vi "map_trap_switch.vi"() -> ()   [LabVIEW 2015]
panel:
  in  "ZeroLaser":bool
  in  "done":bool
  out "Mapping file":string
  in  "Done ?":bool
  in  "KILL":bool
  in  "PAUSE":bool
  in  "RESUME":bool
  in  "QUIT":bool
  in  "up done":bool
  in  "z up":bool
  in  "Done":bool
  in  "z piastra":bool
  in  "x piastra":bool
  in  "goto y pos":bool
  in  "goto x pos":bool
  in  "Panello o pcb?":bool
  in  "End":bool
  in  "zero z - end":bool
  in  "zero x - end":bool
  in  "zero y - end":bool
  in  "positioning done":bool
  out "output":string
  out "command":string
  in  "zero done":bool
  in  "zero z":bool
  in  "zero x":bool
  in  "zero y":bool
  # "Comandi di emergenza"
  # "In alto: TRUE ---> Panello"
  # "In basso: FALSE ---> PCB"
  # "Posiziono in zero"
  # "Vado sulla piastra \ne azzero"
  # "Azzero  il laser"
  # "Alzo il laser"
  # "Vado in posizione"
  # "Ritorno a zero"
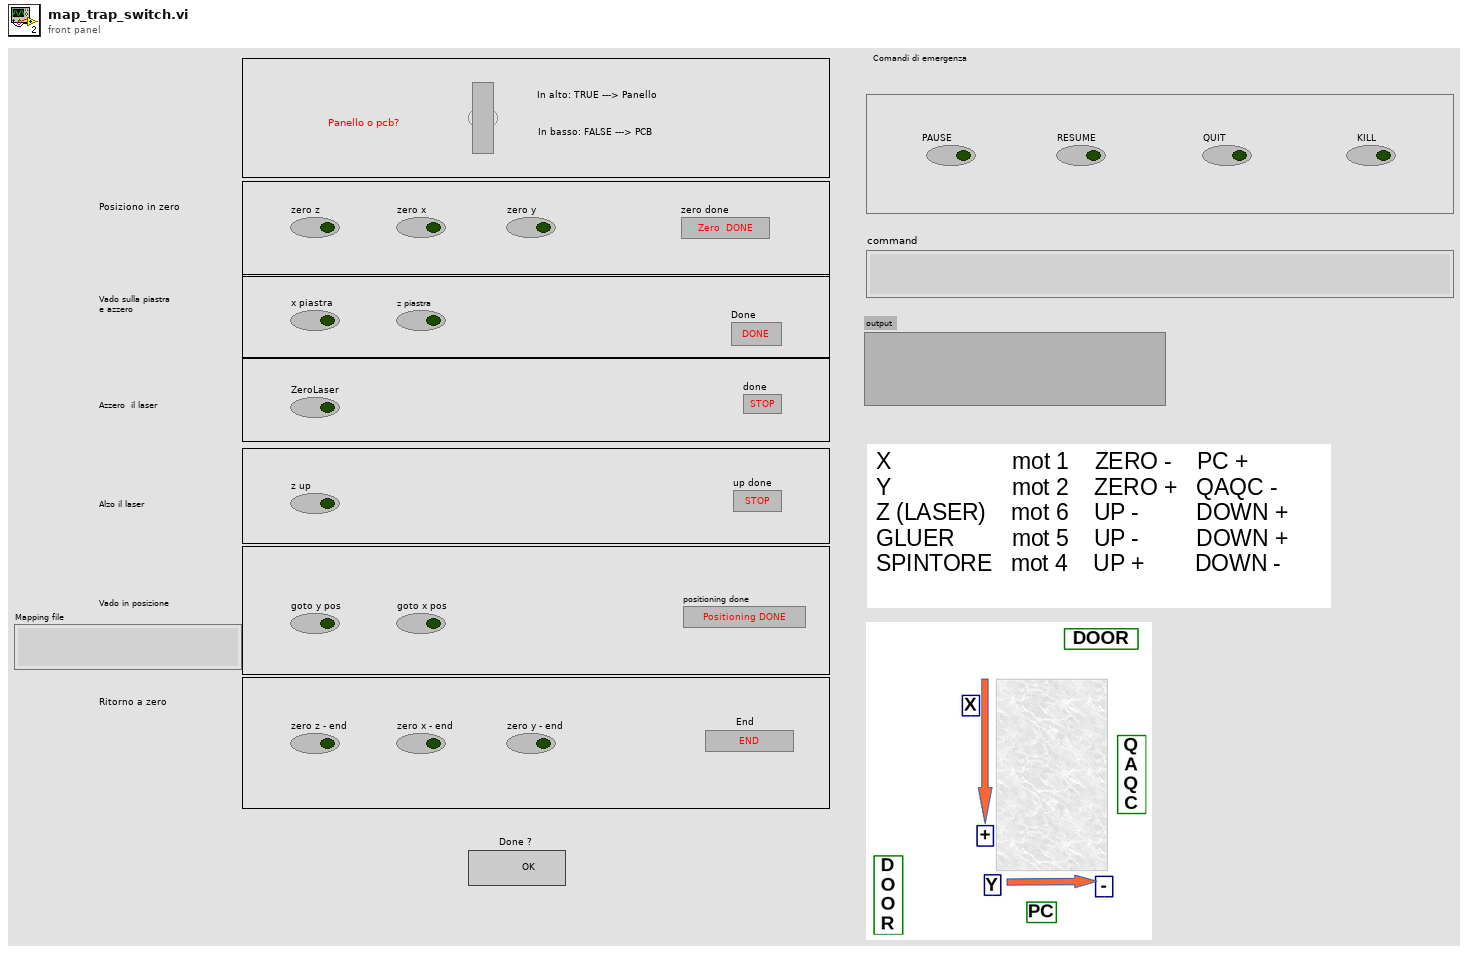
[diagram p1: front panel]
types:
  T1 = enum16{"open", "replace", "create", "open or create", "replace or create", "replace or create with confirmation"}
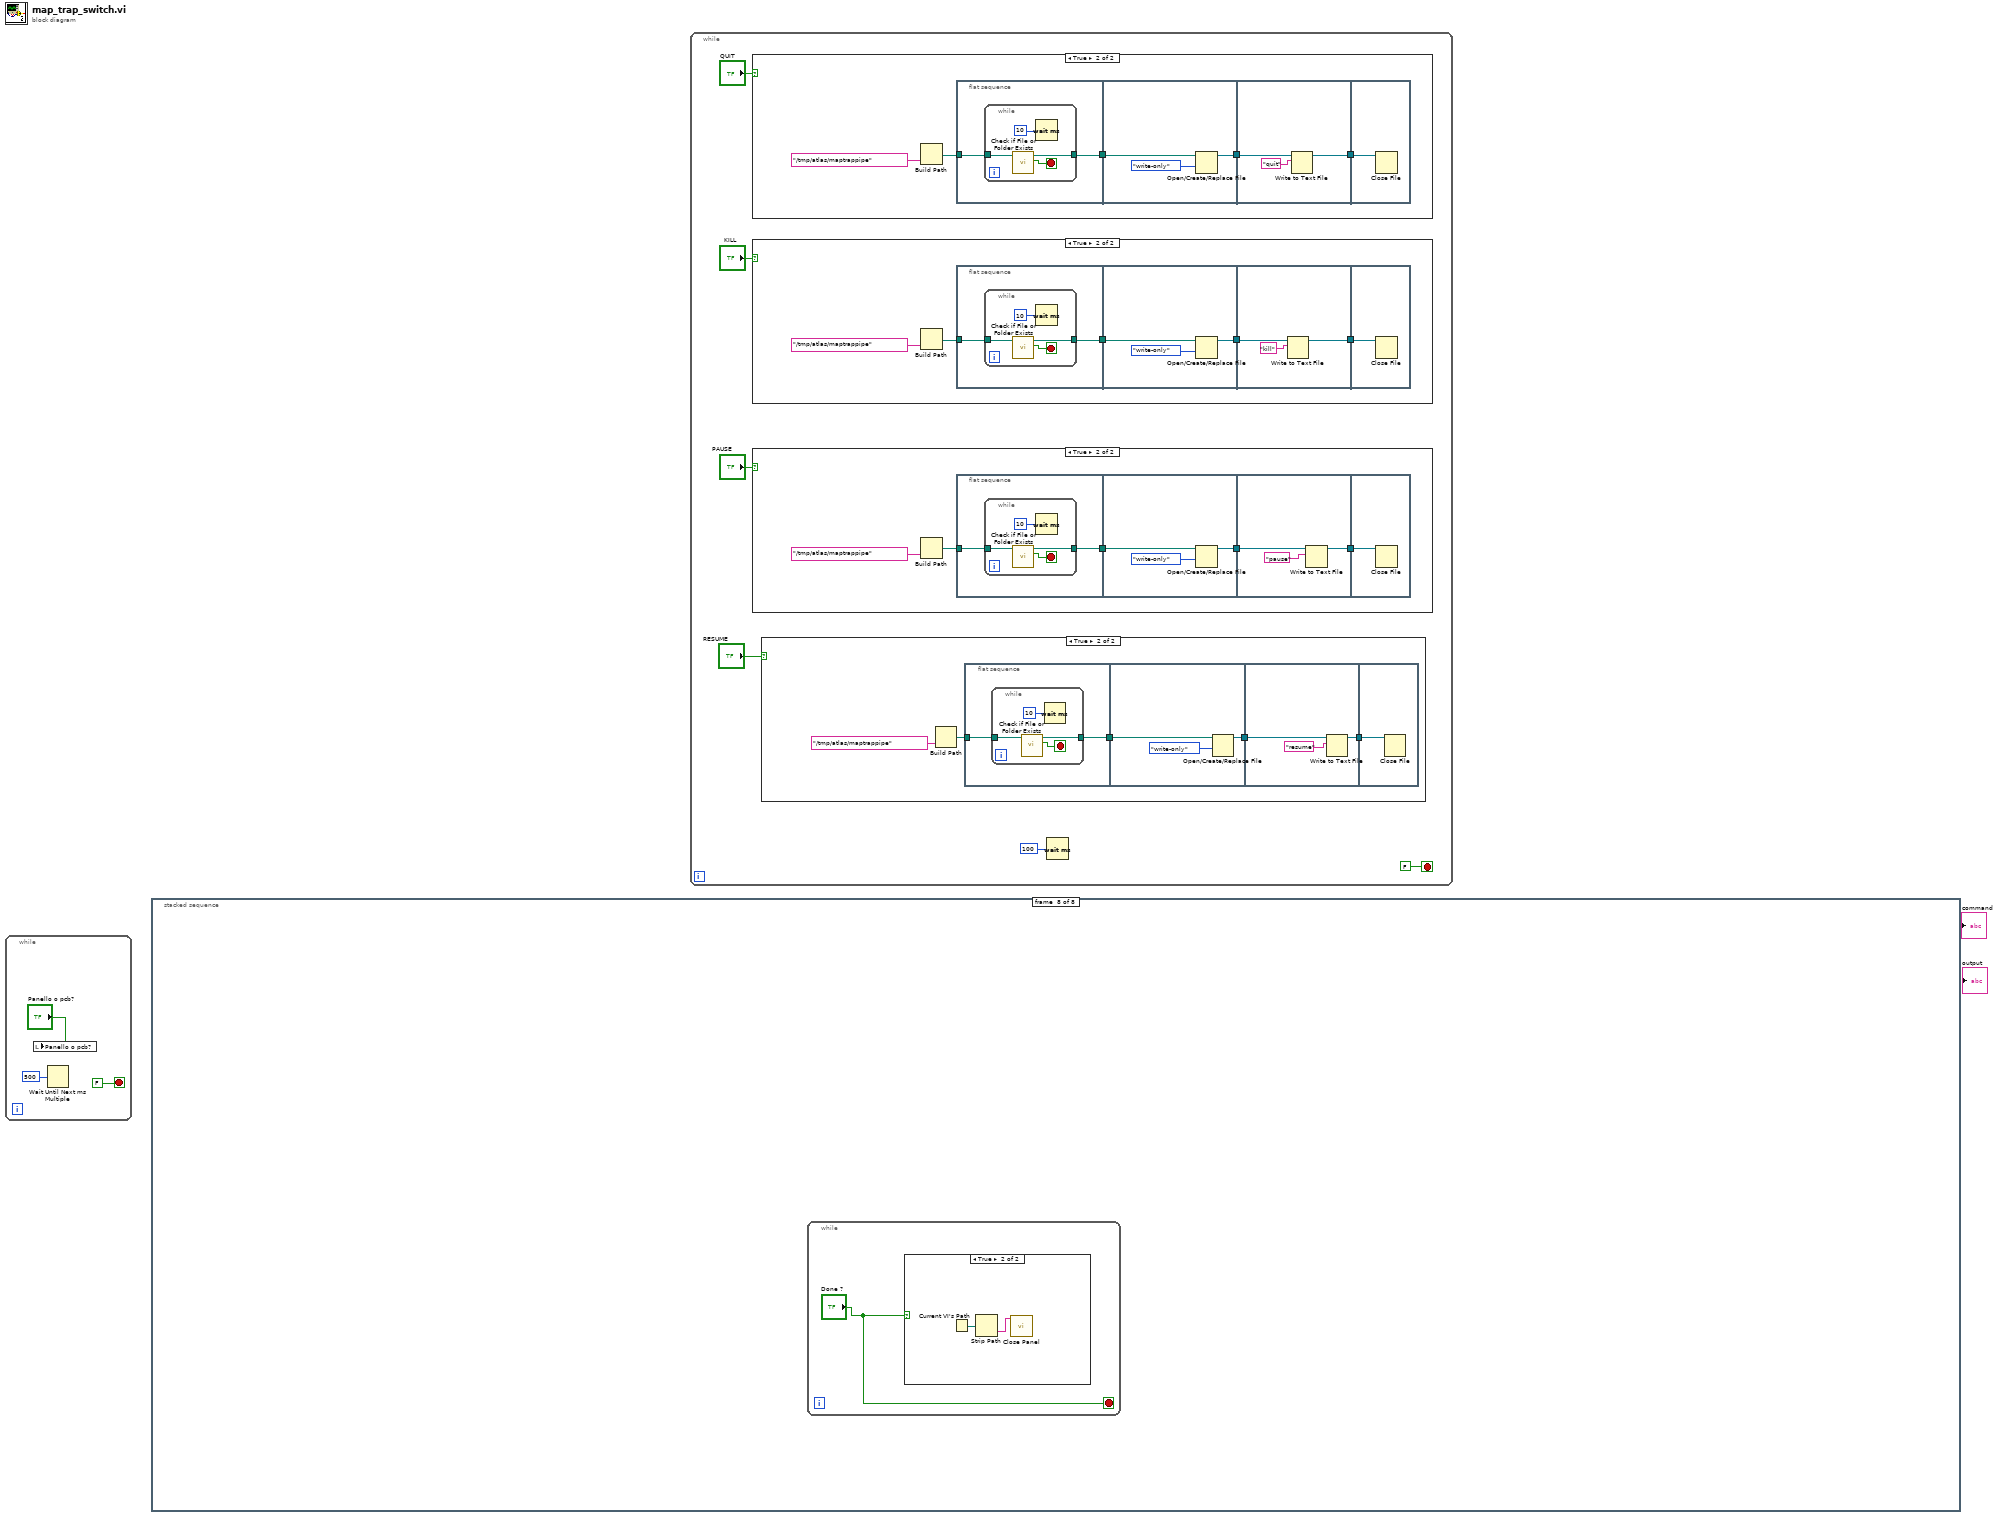
[diagram p0: block diagram]
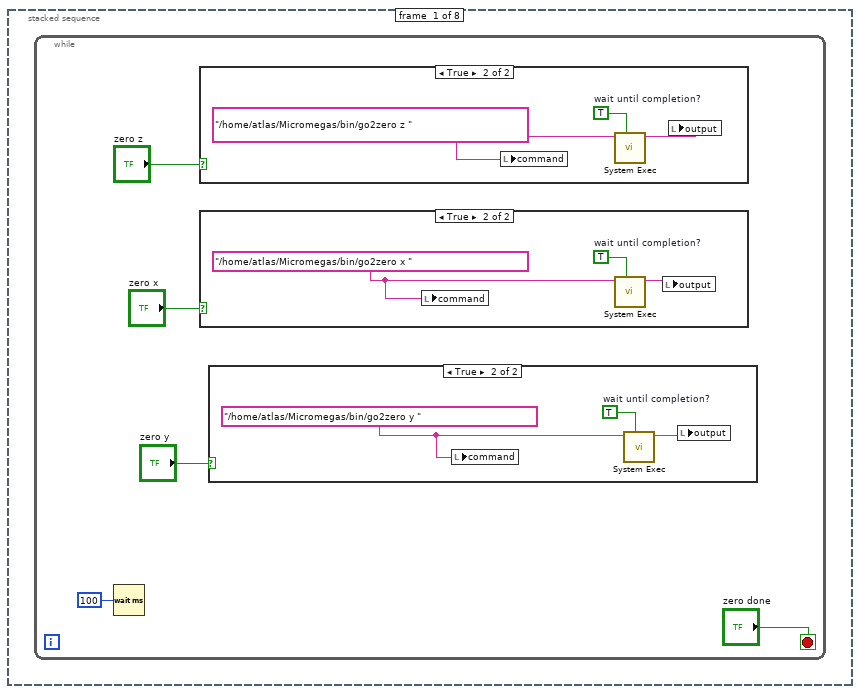
[diagram p6: hidden frame]
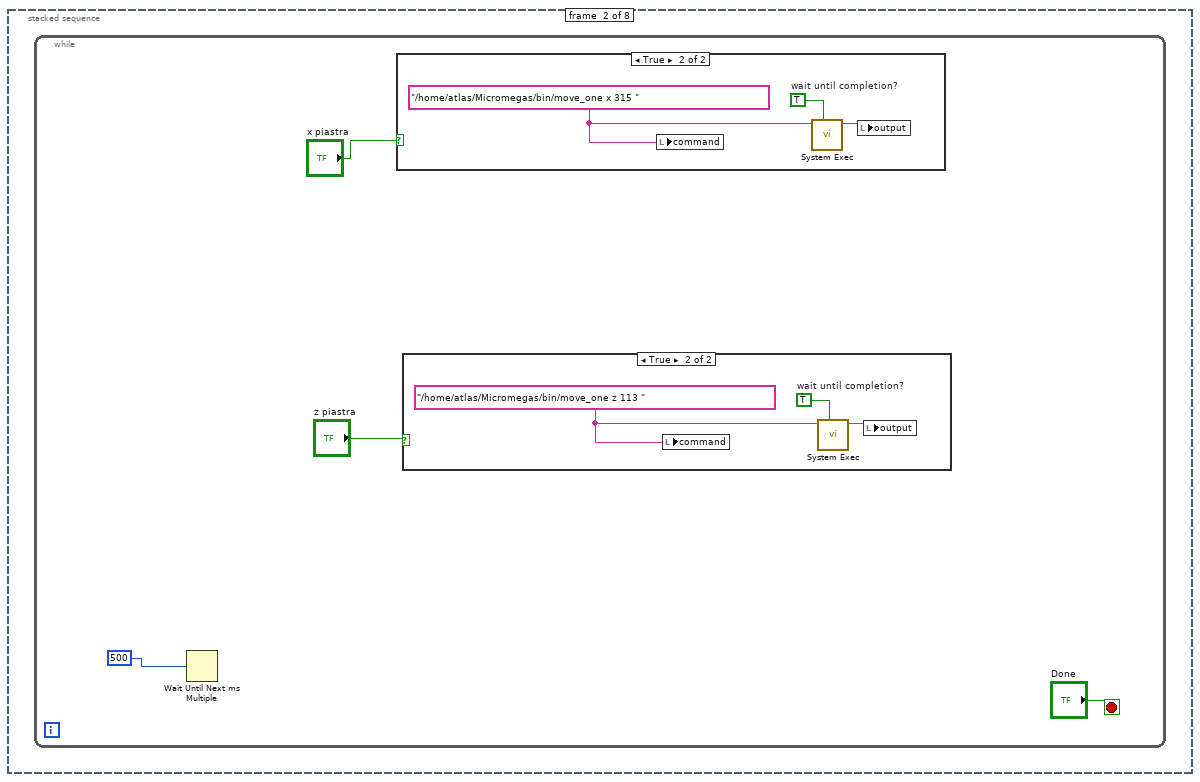
[diagram p10: hidden frame]
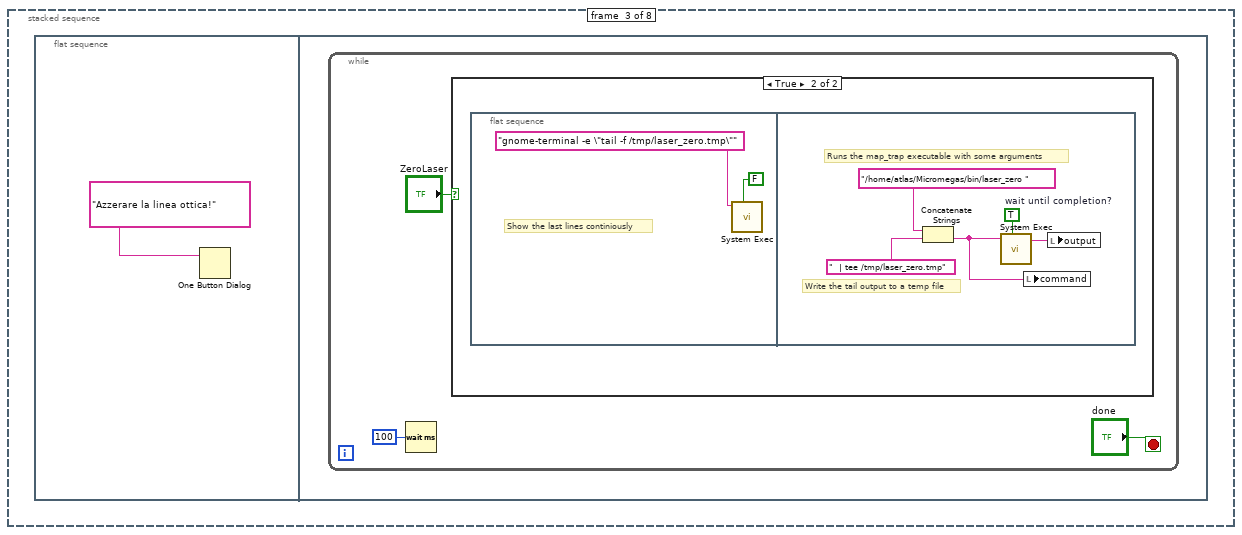
[diagram p13: hidden frame]
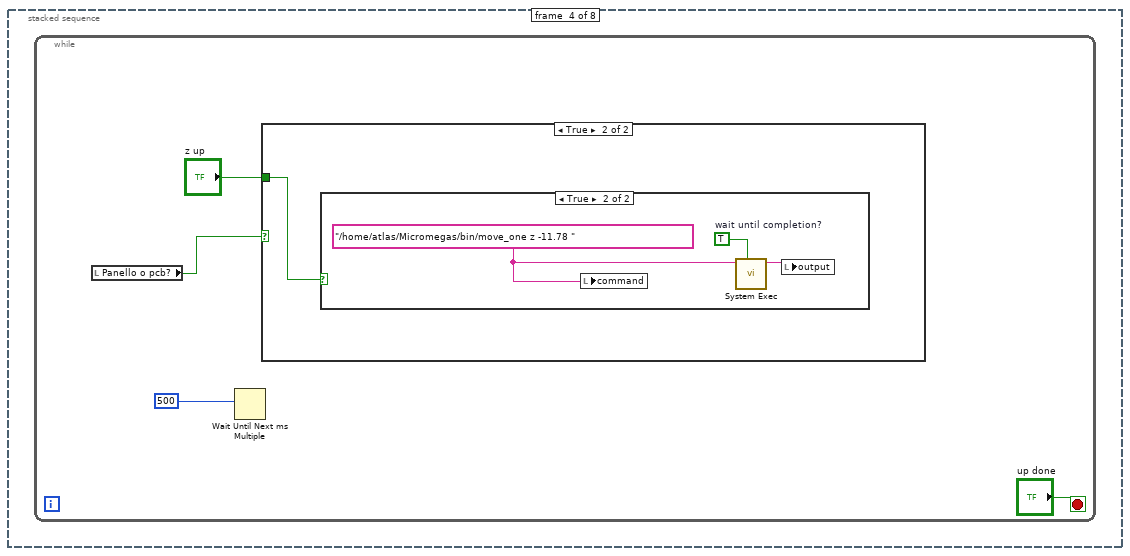
[diagram p15: hidden frame]
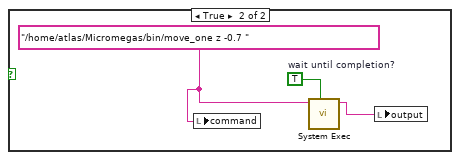
[diagram p17: hidden frame]
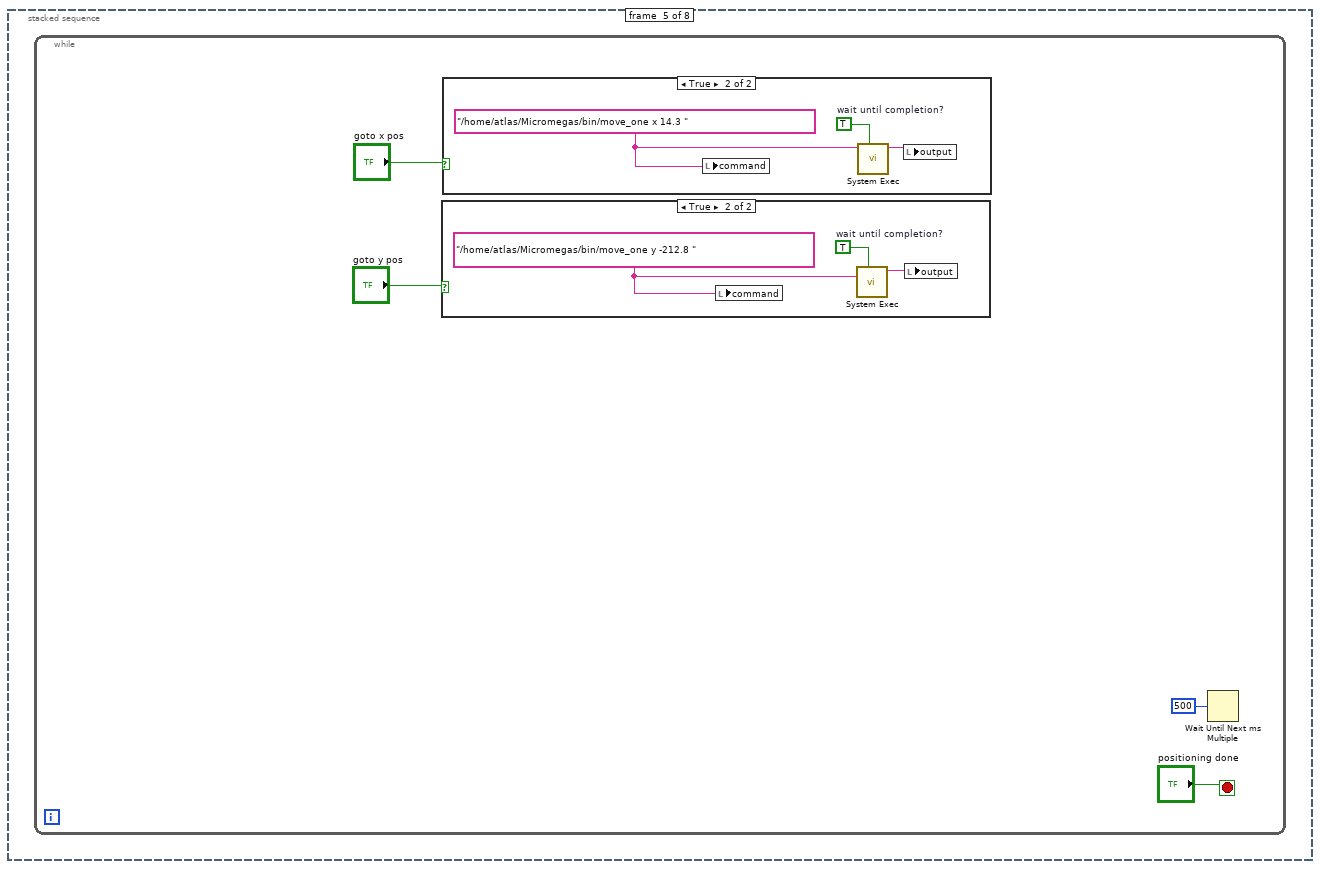
[diagram p19: hidden frame]
diagram:
  n1 = while {
    stop <- FALSE stop-if-true
    n2 = local write "Panello o pcb?"("Panello o pcb?") -> ()
    n3 = Wait Until Next ms Multiple(millisecond multiple=u32 500) -> ()  [unwired: 1 out]
  }
  n4 = stacked-sequence {
    frame #0 {
      n5 = while {
        stop <- "zero done" stop-if-true
        n6 = Wait (ms)(milliseconds to wait=u32 100) -> ()  [unwired: 1 out]
        n7 = case shown="True" "zero z" {
          frame False {
          }
          frame True {
            w16 = "/home/atlas/Micromegas/bin/go2zero z " ("string")
            w17 = TRUE  # wait until completion?
            n8 = local write "command"(w16) -> ()
            n9 = call <vilib>:"System Exec.vi"("wait until completion? (T)"=w17, "command line"=w16) -> ("standard output"=w15:string)  [unwired: 6 in, 3 out]
            n10 = local write "output"(w15) -> ()
          }
        }
        n11 = case shown="True" "zero x" {
          frame False {
          }
          frame True {
            w13 = "/home/atlas/Micromegas/bin/go2zero x " ("string")
            w14 = TRUE  # wait until completion?
            n12 = local write "command"(w13) -> ()
            n13 = call <vilib>:"System Exec.vi"("wait until completion? (T)"=w14, "command line"=w13) -> ("standard output"=w12:string)  [unwired: 6 in, 3 out]
            n14 = local write "output"(w12) -> ()
          }
        }
        n15 = case shown="True" "zero y" {
          frame False {
          }
          frame True {
            w10 = "/home/atlas/Micromegas/bin/go2zero y " ("string")
            w11 = TRUE  # wait until completion?
            n16 = local write "command"(w10) -> ()
            n17 = call <vilib>:"System Exec.vi"("wait until completion? (T)"=w11, "command line"=w10) -> ("standard output"=w9:string)  [unwired: 6 in, 3 out]
            n18 = local write "output"(w9) -> ()
          }
        }
      }
    }
    frame #1 {
      n19 = while {
        stop <- "Done" stop-if-true
        n20 = Wait Until Next ms Multiple(millisecond multiple=u32 500 ("millisecond timer value")) -> ()  [unwired: 1 out]
        n21 = case shown="True" "x piastra" {
          frame False {
          }
          frame True {
            w25 = "/home/atlas/Micromegas/bin/move_one x 315 " ("string")
            w27 = TRUE  # wait until completion?
            n22 = local write "command"(w25) -> ()
            n23 = call <vilib>:"System Exec.vi"("wait until completion? (T)"=w27, "command line"=w25) -> ("standard output"=w26:string)  [unwired: 6 in, 3 out]
            n24 = local write "output"(w26) -> ()
          }
        }
        n25 = case shown="True" "z piastra" {
          frame False {
          }
          frame True {
            w22 = "/home/atlas/Micromegas/bin/move_one z 113 " ("string")
            w24 = TRUE  # wait until completion?
            n26 = local write "command"(w22) -> ()
            n27 = call <vilib>:"System Exec.vi"("wait until completion? (T)"=w24, "command line"=w22) -> ("standard output"=w23:string)  [unwired: 6 in, 3 out]
            n28 = local write "output"(w23) -> ()
          }
        }
      }
    }
    frame #2 {
      n29 = flat-sequence {
        frame #0 {
          n30 = One Button Dialog(message="Azzerare la linea ottica!") -> ()  [unwired: 1 in, 1 out]
        }
        frame #1 {
          n31 = while {
            stop <- "done" stop-if-true
            n32 = Wait (ms)(milliseconds to wait=u32 100) -> ()  [unwired: 1 out]
            n33 = case shown="True" "ZeroLaser" {
              frame False {
              }
              frame True {
                n34 = flat-sequence {
                  frame #0 {
                    # "Show the last lines continiously"
                    n35 = call <vilib>:"System Exec.vi"("wait until completion? (T)"=FALSE, "command line"="gnome-terminal -e \"tail -f /tmp/laser_zero.tmp\"") -> ()  [unwired: 6 in, 4 out]
                  }
                  frame #1 {
                    w34 = TRUE  # wait until completion?
                    # "Write the tail output to a temp file"
                    # "Runs the map_trap executable with some arguments"
                    n36 = Concatenate Strings("/home/atlas/Micromegas/bin/laser_zero " ("string"), "  | tee /tmp/laser_zero.tmp" ("string")) -> (w38:string)
                    n37 = call <vilib>:"System Exec.vi"("wait until completion? (T)"=w34, "command line"=w38) -> ("standard output"=w37:string)  [unwired: 6 in, 3 out]
                    n38 = local write "command"(w38) -> ()
                    n39 = local write "output"(w37) -> ()
                  }
                }
              }
            }
          }
        }
      }
    }
    frame #3 {
      n40 = while {
        stop <- "up done" stop-if-true
        n41 = local read "Panello o pcb?"() -> (w40:bool)
        n42 = Wait Until Next ms Multiple(millisecond multiple=u32 500 ("millisecond timer value")) -> ()  [unwired: 1 out]
        n43 = case shown="True" w40 {
          tunnel: "z up" -> [w43 w47]
          frame False {
            n44 = case shown="False" w43 {
              frame False {
              }
              frame True {
                w46 = TRUE  # wait until completion?
                w45 = "/home/atlas/Micromegas/bin/move_one z -0.7 " ("string")
                n45 = local write "command"(w45) -> ()
                n46 = call <vilib>:"System Exec.vi"("wait until completion? (T)"=w46, "command line"=w45) -> ("standard output"=w44:string)  [unwired: 6 in, 3 out]
                n47 = local write "output"(w44) -> ()
              }
            }
          }
          frame True {
            n48 = case shown="True" w47 {
              frame False {
              }
              frame True {
                w48 = "/home/atlas/Micromegas/bin/move_one z -11.78 " ("string")
                w50 = TRUE  # wait until completion?
                n49 = local write "command"(w48) -> ()
                n50 = call <vilib>:"System Exec.vi"("wait until completion? (T)"=w50, "command line"=w48) -> ("standard output"=w49:string)  [unwired: 6 in, 3 out]
                n51 = local write "output"(w49) -> ()
              }
            }
          }
        }
      }
    }
    frame #4 {
      n52 = while {
        stop <- "positioning done" stop-if-true
        n53 = case shown="True" "goto y pos" {
          frame False {
          }
          frame True {
            w55 = "/home/atlas/Micromegas/bin/move_one y -212.8 " ("string")
            w57 = TRUE  # wait until completion?
            n54 = local write "command"(w55) -> ()
            n55 = call <vilib>:"System Exec.vi"("wait until completion? (T)"=w57, "command line"=w55) -> ("standard output"=w56:string)  [unwired: 6 in, 3 out]
            n56 = local write "output"(w56) -> ()
          }
        }
        n57 = case shown="True" "goto x pos" {
          frame False {
          }
          frame True {
            w58 = "/home/atlas/Micromegas/bin/move_one x 14.3 " ("string")
            w60 = TRUE  # wait until completion?
            n58 = local write "command"(w58) -> ()
            n59 = call <vilib>:"System Exec.vi"("wait until completion? (T)"=w60, "command line"=w58) -> ("standard output"=w59:string)  [unwired: 6 in, 3 out]
            n60 = local write "output"(w59) -> ()
          }
        }
        n61 = Wait Until Next ms Multiple(millisecond multiple=u32 500) -> ()  [unwired: 1 out]
      }
    }
    frame #5 {
      n62 = flat-sequence {
        frame #0 {
          # "Show the last lines continiously"
          n63 = Open/Create/Replace File(file path (use dialog)=path "/tmp/map_trap_laser_step.tmp", operation (0:open)=T1."open or create") -> ()  [unwired: 4 in, 3 out]
          n64 = call <vilib>:"System Exec.vi"("wait until completion? (T)"=FALSE, "command line"="gnome-terminal -e \"tail -f /tmp/map_trap_laser_step.tmp\"") -> ()  [unwired: 6 in, 4 out]
        }
        frame #1 {
          w71 = TRUE  # wait until completion?
          # "need to chose table/stiffback"
          # "Write the tail output to a temp file"
          # "Runs the map_trap executable with some arguments"
          # "W: x length, y length\nX: x step, x speed\nY: y step, y speed\nT: z step, z speed"
          n65 = Concatenate Strings("/home/atlas/Micromegas/bin/map_trap_laser_step  " ("string"), "" ("string"), "-w 2100 1000 -x 100 20 -y 100 20 -i 0" ("string"), "  | tee /tmp/map_trap_laser_step.tmp" ("string")) -> (w66:string)
          n66 = local write "command"(w66) -> ()
          n67 = call <vilib>:"System Exec.vi"("wait until completion? (T)"=w71, "command line"=w66) -> ("standard output"=w65:string)  [unwired: 6 in, 3 out]
          n68 = local write "output"(w65) -> ()
        }
        frame #2 {
          n69 = call <vilib>:"Get System Directory.vi"("system directory type"=0) -> ("system directory"=w73:path)  [unwired: 10 in]
          n70 = Build Path(base path=w73, name or relative path="Micromegas/ProdData/mapping/map_trap_filename.txt") -> (appended path=w72:path)
          n71 = Open/Create/Replace File(file path (use dialog)=w72, operation (0:open)=T1."open") -> (refnum out=w78:refnum<file>, error out=w77:errorcluster)  [unwired: 4 in, 1 out]
          n72 = Read from Text File(file (use dialog)=w78, error in=w77) -> (text=→"Mapping file":string)  [unwired: 2 in, 3 out]
        }
      }
    }
    frame #6 {
      n73 = while {
        stop <- "End" stop-if-true
        n74 = Wait (ms)(milliseconds to wait=u32 100) -> ()  [unwired: 1 out]
        n75 = case shown="True" "zero z - end" {
          frame False {
          }
          frame True {
            w92 = "/home/atlas/Micromegas/bin/go2zero z " ("string")
            w93 = TRUE  # wait until completion?
            n76 = local write "command"(w92) -> ()
            n77 = call <vilib>:"System Exec.vi"("wait until completion? (T)"=w93, "command line"=w92) -> ("standard output"=w91:string)  [unwired: 6 in, 3 out]
            n78 = local write "output"(w91) -> ()
          }
        }
        n79 = case shown="True" "zero x - end" {
          frame False {
          }
          frame True {
            w89 = "/home/atlas/Micromegas/bin/go2zero x " ("string")
            w90 = TRUE  # wait until completion?
            n80 = local write "command"(w89) -> ()
            n81 = call <vilib>:"System Exec.vi"("wait until completion? (T)"=w90, "command line"=w89) -> ("standard output"=w88:string)  [unwired: 6 in, 3 out]
            n82 = local write "output"(w88) -> ()
          }
        }
        n83 = case shown="True" "zero y - end" {
          frame False {
          }
          frame True {
            w86 = "/home/atlas/Micromegas/bin/go2zero y " ("string")
            w87 = TRUE  # wait until completion?
            n84 = local write "command"(w86) -> ()
            n85 = call <vilib>:"System Exec.vi"("wait until completion? (T)"=w87, "command line"=w86) -> ("standard output"=w85:string)  [unwired: 6 in, 3 out]
            n86 = local write "output"(w85) -> ()
          }
        }
      }
    }
    frame #7 {
      n87 = while {
        stop <- "Done ?" stop-if-true
        n88 = case shown="True" "Done ?" {
          frame False {
          }
          frame True {
            n89 = Current VI's Path() -> (path=w95:path)
            n90 = Strip Path(path=w95) -> (name=w96:string)  [unwired: 1 out]
            n91 = call <vilib>:"Close Panel.vi"("VI name"=w96) -> ()  [unwired: 10 in, 1 out]
          }
        }
      }
    }
  }
  n92 = while {
    stop <- FALSE stop-if-true
    n93 = case shown="True" "QUIT" {
      frame False {
      }
      frame True {
        n94 = Build Path(name or relative path="/tmp/atlas/maptrappipe" ("string")) -> (appended path=w157:path)  [unwired: 1 in]
        n95 = flat-sequence {
          tunnel: [w163] -> w161
          tunnel: w157 -> [w162]
          tunnel: w161 -> [w170]
          tunnel: [w168] -> w160
          tunnel: w160 -> [w173]
          tunnel: [w172] -> w159
          tunnel: w159 -> [w174]
          frame #0 {
            n96 = while {
              tunnel: [w165] -> w163
              tunnel: w162 -> [w164]
              stop <- w166 stop-if-true
              n97 = call <vilib>:"Check if File or Folder Exists.vi"("path"=w164) -> ("file or folder exists?"=w166:bool, "dup path"=w165:path)  [unwired: 8 in, 1 out]
              n98 = Wait (ms)(milliseconds to wait=u32 10) -> ()  [unwired: 1 out]
            }
          }
          frame #1 {
            n99 = Open/Create/Replace File(file path (use dialog)=w170, access (0:read/write)=enum16{"read/write", "read-only", "write-only"}."write-only") -> (refnum out=w168:refnum<file>)  [unwired: 4 in, 2 out]
          }
          frame #2 {
            n100 = Write to Text File(file (use dialog)=w173, text="quit") -> (refnum out=w172:refnum<file>)  [unwired: 2 in, 2 out]
          }
          frame #3 {
            n101 = Close File(refnum=w174) -> ()  [unwired: 1 in, 2 out]
          }
        }
      }
    }
    n102 = case shown="True" "KILL" {
      frame False {
      }
      frame True {
        n103 = Build Path(name or relative path="/tmp/atlas/maptrappipe" ("string")) -> (appended path=w121:path)  [unwired: 1 in]
        n104 = flat-sequence {
          tunnel: [w127] -> w125
          tunnel: w121 -> [w126]
          tunnel: w125 -> [w134]
          tunnel: [w132] -> w124
          tunnel: w124 -> [w137]
          tunnel: [w136] -> w123
          tunnel: w123 -> [w138]
          frame #0 {
            n105 = while {
              tunnel: [w129] -> w127
              tunnel: w126 -> [w128]
              stop <- w130 stop-if-true
              n106 = call <vilib>:"Check if File or Folder Exists.vi"("path"=w128) -> ("file or folder exists?"=w130:bool, "dup path"=w129:path)  [unwired: 8 in, 1 out]
              n107 = Wait (ms)(milliseconds to wait=u32 10) -> ()  [unwired: 1 out]
            }
          }
          frame #1 {
            n108 = Open/Create/Replace File(file path (use dialog)=w134, access (0:read/write)=enum16{"read/write", "read-only", "write-only"}."write-only") -> (refnum out=w132:refnum<file>)  [unwired: 4 in, 2 out]
          }
          frame #2 {
            n109 = Write to Text File(file (use dialog)=w137, text="kill") -> (refnum out=w136:refnum<file>)  [unwired: 2 in, 2 out]
          }
          frame #3 {
            n110 = Close File(refnum=w138) -> ()  [unwired: 1 in, 2 out]
          }
        }
      }
    }
    n111 = case shown="True" "PAUSE" {
      frame False {
      }
      frame True {
        n112 = Build Path(name or relative path="/tmp/atlas/maptrappipe" ("string")) -> (appended path=w103:path)  [unwired: 1 in]
        n113 = flat-sequence {
          tunnel: [w109] -> w107
          tunnel: w103 -> [w108]
          tunnel: w107 -> [w116]
          tunnel: [w114] -> w106
          tunnel: w106 -> [w119]
          tunnel: [w118] -> w105
          tunnel: w105 -> [w120]
          frame #0 {
            n114 = while {
              tunnel: [w111] -> w109
              tunnel: w108 -> [w110]
              stop <- w112 stop-if-true
              n115 = call <vilib>:"Check if File or Folder Exists.vi"("path"=w110) -> ("file or folder exists?"=w112:bool, "dup path"=w111:path)  [unwired: 8 in, 1 out]
              n116 = Wait (ms)(milliseconds to wait=u32 10) -> ()  [unwired: 1 out]
            }
          }
          frame #1 {
            n117 = Open/Create/Replace File(file path (use dialog)=w116, access (0:read/write)=enum16{"read/write", "read-only", "write-only"}."write-only") -> (refnum out=w114:refnum<file>)  [unwired: 4 in, 2 out]
          }
          frame #2 {
            n118 = Write to Text File(file (use dialog)=w119, text="pause") -> (refnum out=w118:refnum<file>)  [unwired: 2 in, 2 out]
          }
          frame #3 {
            n119 = Close File(refnum=w120) -> ()  [unwired: 1 in, 2 out]
          }
        }
      }
    }
    n120 = case shown="True" "RESUME" {
      frame False {
      }
      frame True {
        n121 = Build Path(name or relative path="/tmp/atlas/maptrappipe" ("string")) -> (appended path=w139:path)  [unwired: 1 in]
        n122 = flat-sequence {
          tunnel: [w145] -> w143
          tunnel: w139 -> [w144]
          tunnel: w143 -> [w152]
          tunnel: [w150] -> w142
          tunnel: w142 -> [w155]
          tunnel: [w154] -> w141
          tunnel: w141 -> [w156]
          frame #0 {
            n123 = while {
              tunnel: [w147] -> w145
              tunnel: w144 -> [w146]
              stop <- w148 stop-if-true
              n124 = call <vilib>:"Check if File or Folder Exists.vi"("path"=w146) -> ("file or folder exists?"=w148:bool, "dup path"=w147:path)  [unwired: 8 in, 1 out]
              n125 = Wait (ms)(milliseconds to wait=u32 10) -> ()  [unwired: 1 out]
            }
          }
          frame #1 {
            n126 = Open/Create/Replace File(file path (use dialog)=w152, access (0:read/write)=enum16{"read/write", "read-only", "write-only"}."write-only") -> (refnum out=w150:refnum<file>)  [unwired: 4 in, 2 out]
          }
          frame #2 {
            n127 = Write to Text File(file (use dialog)=w155, text="resume") -> (refnum out=w154:refnum<file>)  [unwired: 2 in, 2 out]
          }
          frame #3 {
            n128 = Close File(refnum=w156) -> ()  [unwired: 1 in, 2 out]
          }
        }
      }
    }
    n129 = Wait (ms)(milliseconds to wait=100) -> ()  [unwired: 1 out]
  }
